vi "Format Date to String.vi"(9 "Month":T1, 11 "YYYY":i32) -> (2 "Year-Mo":string)   [LabVIEW 2018, in "Account History.lvclass"]
uses:
  Account History.lvclass
  Month.ctl
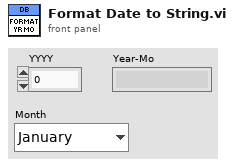
[diagram p1: front panel]
types:
  T1 = typedef "Account History.lvclass/Month.ctl" = enum16{"January", "February", "March", "April", "May", "June", "July", "August", "September", "October", "November", "December"}
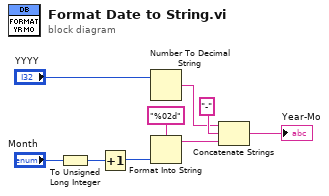
[diagram p0: block diagram]
diagram:
  n1 = To Unsigned Long Integer(number="Month") -> (unsigned 32bit integer=w2:u32)
  n2 = Increment(x=w2) -> (x+1=w1:u32)
  n3 = Number To Decimal String(number="YYYY") -> (decimal integer string=w4:string)  [unwired: 1 in]
  n4 = Format Into String(format string="%02d" ("string"), w1) -> (resulting string=w6:string)  [unwired: 2 in, 1 out]
  n5 = Concatenate Strings(w4, "-" ("string"), w6) -> (→"Year-Mo":string)
